vi "High Throughput Streaming (FPGA) PXIe-796xR.vi"() -> ()   [LabVIEW 2016]
doc: "Example Description:\nThis FPGA VI has two data streaming engines. One to stream data to disk from the FPGA and one to stream data from disk to the FPGA. The throughput of the streams is controled by accessing the DMA FIFOs on a subset of the cycles of the SCTLs.\n\nRunning the VI:\nThis VI m ust be run from one of the High Throughput Streaming - XXXXXXX (Host).vi files in the project. Refer to the host documentation for steps regarding running and configuring this FPGA VI.\n\nExecution Steps:\nRefer to teh block diagram of this VI for excution comments."
uses:
  <vilib>/Platform/TimedLoop/XDataNode/timing_clust.ctl
  <vilib>/Platform/TimedLoop/XDataNode/nitl_modes.ctl
  <vilib>/Platform/TimedLoop/XDataNode/wakeup.ctl
  <vilib>/rvi/Emulation/niFpgaGetClockAttributes.vi
  <vilib>/rvi/Emulation/niFpgaSctlEmulationGetInTimedLoop.vi
  <vilib>/rvi/Emulation/niFpgaEmulationReportErrorSimple.vi
  <vilib>/rvi/Emulation/niFpgaCriticalErrorInLSC.vi
  <vilib>/rvi/interface/RandomDataEmulation/nirviRandomDataMultiElementFPGAFIFO.vi
  <instcachedir>/0/nirviRandomDataMultiElementFPGAFIFO_6740B454F3C245F78F76ED91F73FD8DB.lvgen/nirviRandomDataMultiElementFPGAFIFO_6740B454F3C245F78F76ED91F73FD8DB_001.vi
  <vilib>/rvi/interface/RandomDataEmulation/niFpgaRandomDataHandleErrors.vi
  <vilib>/Platform/TimedLoop/XDataNode/XDataNode.xnode
  <vilib>/rvi/DataTransferAndStorage/Container/XNode/niFpgaContainer.xnode
  <vilib>/rvi/interface/RandomDataEmulation/nirviRandomDataFpgaMultiElementTemplate.vi
  <vilib>/Platform/TimedLoop/XDataNode/XDNodeRunTimeDep.lvlib
panel:
  in  "output.Requested Throughput Denominator":u16=200
  in  "input.Requested Throughput Denominator":u16=200
  out "input.Max Throughput":u16
  in  "input.Requested Throughput":u16
  out "input.FIFO Transfer Status":T1
  in  "output.Requested Throughput":u16
  out "output.Max Throughput":u16
  out "output.FIFO Transfer Status":T2
  in  "output.Start":bool
  out "output.Ever Timed Out?":bool
  in  "output.Reset":bool
  out "output.Number of Elements to Read":u32
  out "output.Minimum Number of Elements to Read":u32
  out "output.FIFO Size":u32
  in  "output.Stop":bool
  in  "input.Stop":bool
  in  "input.Start":bool
  out "input.FIFO Size":u32
  out "input.Minimum Number of Elements to Write":u32
  out "input.Number of Elements to Write":u32
  in  "input.Reset":bool
  out "input.Ever Timed Out?":bool
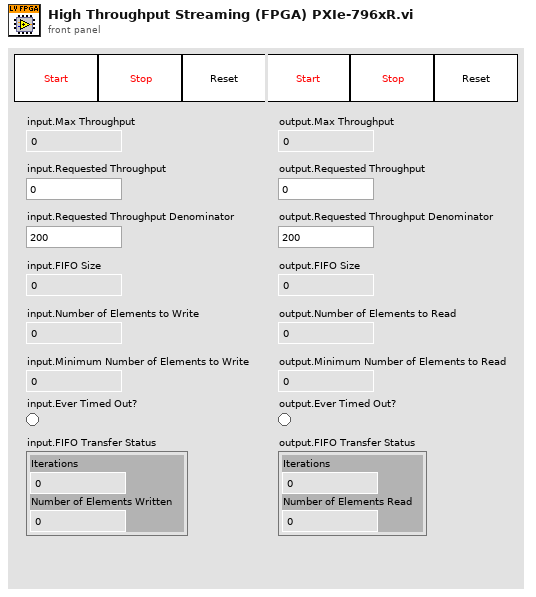
[diagram p1: front panel]
types:
  T1 = cluster{"Iterations":u64, "Number of Elements Written":u64}
  T2 = cluster{"Iterations":u64, "Number of Elements Read":u64}
  T3 = typedef "XDNodeRunTimeDep.lvlib/timing_clust.ctl" = cluster{"Expected End [f-1]":u64, "Actual End [f-1]":u64, "Finished Late? [f-1]":bool, "Expected End [i-1]":u64, "Actual End [i-1]":u64, "Finished Late? [i-1]":bool, "Expected Start [i]":u64, "Actual Start [i]":u64, "Expected Start [f]":u64, "Actual Start [f]":u64, "Source Name":string, "Structure Name":string, "Period":i64, "Deadline":i64, "Offset":i64, "Start":i64, "Priority":i32, "Timeout":i32, "Mode":T4, "Wakeup Reason":T5, "Error":errorcluster, "Source Type":string, "Secondary Source Type":string, "Global End Time":u64, "Global Start Time":u64, "Frame Duration":u64, "Iteration Duration":u64, "Assigned CPU":i32, "I/O Scan Engine Mode":u32}
  T4 = typedef "XDNodeRunTimeDep.lvlib/nitl_modes.ctl" = enum32{"No Change", "Process missed periods, maintain original phase", "Discard missed periods, maintain original phase", "Process missed periods, ignore original phase", "Discard missed periods, ignore original phase"}
  T5 = typedef "XDNodeRunTimeDep.lvlib/wakeup.ctl" = enum32{"Normal", "Aborted", "Asynchronous wakeup", "Timing source error", "Timed loop error", "Timeout"}
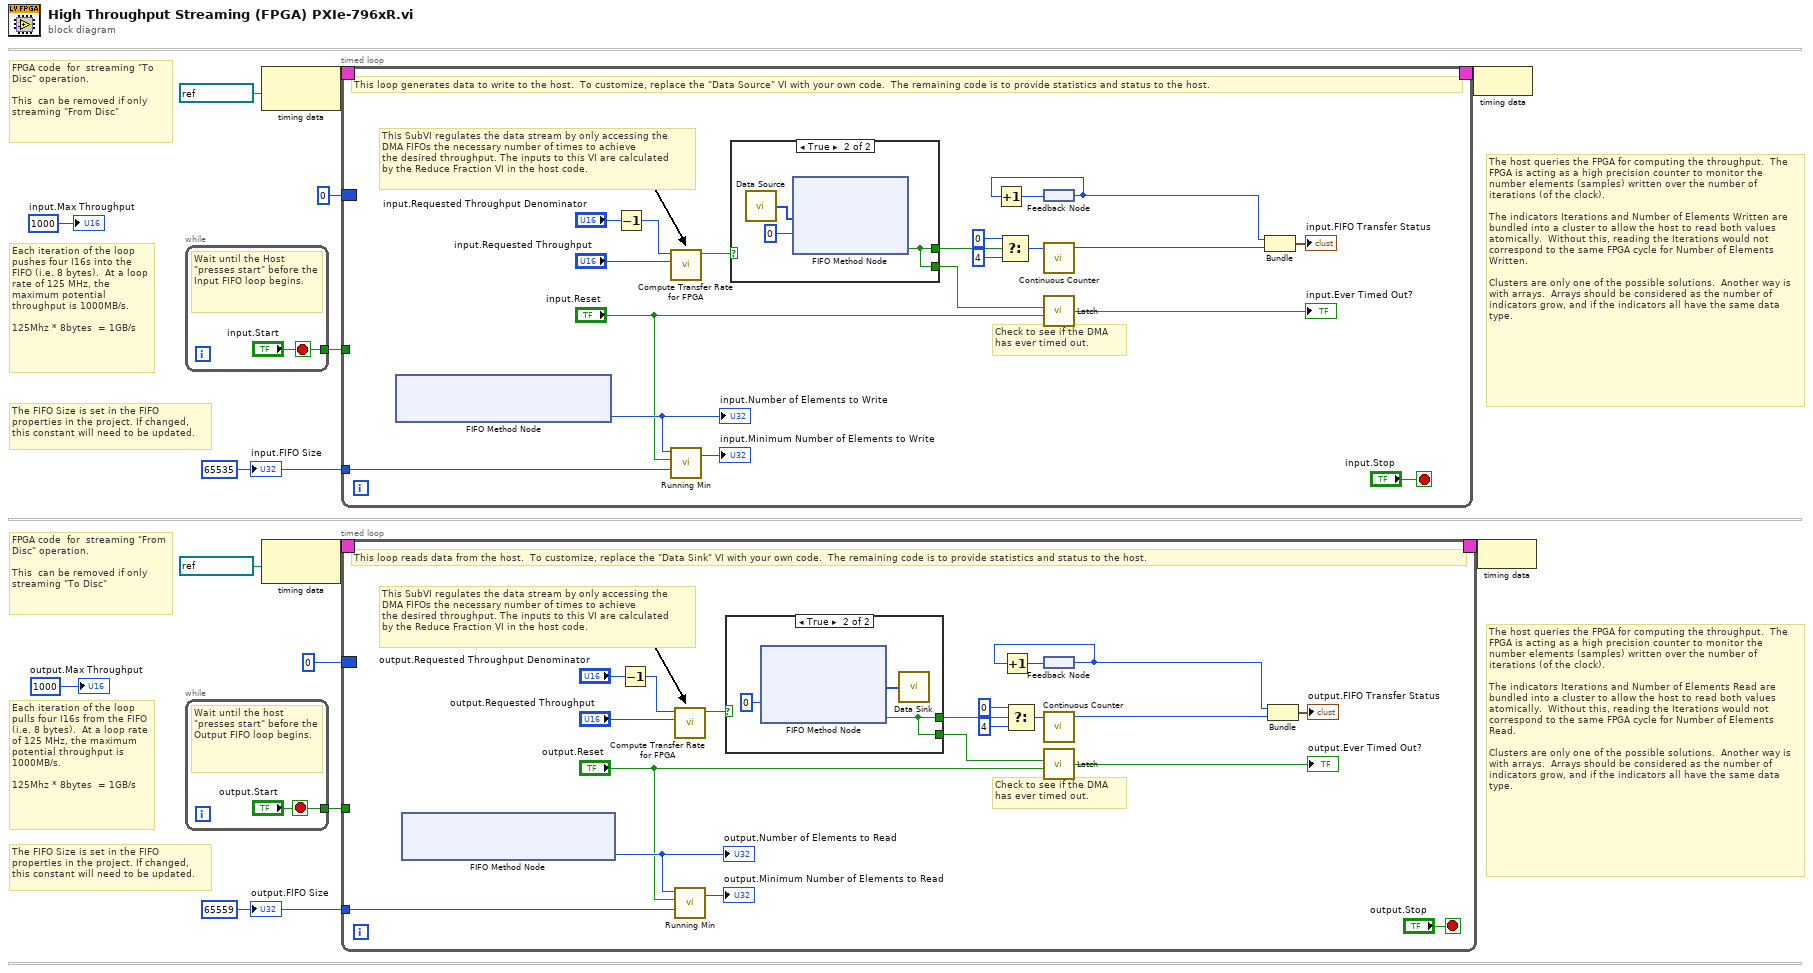
[diagram p0: block diagram]
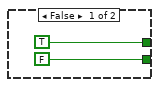
[diagram p2: hidden frame]
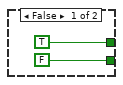
[diagram p3: hidden frame]
diagram:
  w5 = u32 65559 ("output.FIFO Size")
  w2 = u32 65535 ("input.FIFO Size")
  # "The FIFO Size is set in the FIFO\nproperties in the project. If changed, \nthis constant will need to be updated."
  # "The FIFO Size is set in the FIFO\nproperties in the project. If changed, \nthis constant will need to be updated."
  # "FPGA code  for  streaming \"To Disc\" operation. \n\nThis  can be removed if only streaming \"From Disc\""
  # "FPGA code  for  streaming \"From Disc\" operation. \n\nThis  can be removed if only streaming \"To Disc\""
  # "Each iteration of the loop pulls four I16s from the FIFO (i.e. 8 bytes).  At a loop rate of 125 MHz, the maximum potential throughput is 1000MB/s.\n\n125Mhz * 8bytes  = 1GB/s"
  # "The host queries the FPGA for computing the throughput.  The FPGA is acting as a high precision counter to monitor the number elements (samples) written over the number of iterations (of the clock).\n\nThe indicators Iterations and Number of Elements Read are bundled into a cluster to allow the host to read both values atomically.  Without this, reading the Iterations would not correspond to the same FPGA cycle for Number of Elements Read.\n\nClusters are only one of the possible solutions.  Another way is with arrays.  Arrays should be considered as the number of indicators grow, and if the indicators all have the same data type."
  # "Each iteration of the loop pushes four I16s into the FIFO (i.e. 8 bytes).  At a loop rate of 125 MHz, the maximum potential throughput is 1000MB/s.\n\n125Mhz * 8bytes  = 1GB/s"
  # "The host queries the FPGA for computing the throughput.  The FPGA is acting as a high precision counter to monitor the number elements (samples) written over the number of iterations (of the clock).\n\nThe indicators Iterations and Number of Elements Written are bundled into a cluster to allow the host to read both values atomically.  Without this, reading the Iterations would not correspond to the same FPGA cycle for Number of Elements Written.\n\nClusters are only one of the possible solutions.  Another way is with arrays.  Arrays should be considered as the number of indicators grow, and if the indicators all have the same data type."
  n1 = while {
    tunnel: ["input.Start"] -> w11
    stop <- "input.Start" stop-if-true
    # "Wait until the Host \"presses start\" before the Input FIFO loop begins."
  }
  n2 = while {
    tunnel: ["output.Start"] -> w8
    stop <- "output.Start" stop-if-true
    # "Wait until the host \"presses start\" before the Output FIFO loop begins."
  }
  n3 = node-c288(refnum<k21> "125 MHz" ("Source Name")) -> (w14:T3)
  n4 = node-c288(refnum<k21> "125 MHz" ("Source Name")) -> (w10:T3)
  n5 = timed-loop {
    timing: w14 -> [_]
    timing-out: [_] -> w13
    tunnel: w11 -> [_]
    tunnel: w2 -> [w35]
    border: u64 0 -> [_]
    stop <- "input.Stop" stop-if-true
    # "Check to see if the DMA \nhas ever timed out."
    # "This SubVI regulates the data stream by only accessing the \nDMA FIFOs the necessary number of times to achieve \nthe desired throughput. The inputs to this VI are calculated \nby the Reduce Fraction VI in the host code."
    # "This loop generates data to write to the host.  To customize, replace the \"Data Source\" VI with your own code.  The remaining code is to provide statistics and status to the host."
    n6 = xnode ("FIFO Method Node")() -> ("Number of Elements to Write"=w32:u32)  [unwired: 1 in, 1 out]
    "input.Number of Elements to Write" <- w32
    n7 = Decrement(x="input.Requested Throughput Denominator") -> (x-1=w18:u16)
    n8 = call "Compute Transfer Rate for FPGA.vi"("Duty Rate"="input.Requested Throughput", "Clock Rate (minus 1)"=w18) -> ("Output"=w21:bool)  [unwired: 4 in, 1 out]
    n9 = call "Running Min.vi"("Starting Min"=w35, "Reset"="input.Reset", "Next Value"=w32) -> ("Running Min"=→"input.Minimum Number of Elements to Write":u32)  [unwired: 4 in]
    n10 = case shown="True" w21 {
      tunnel: [TRUE ("Timed Out?") w38] -> w20
      tunnel: [FALSE ("Timed Out?") w38] -> w19
      frame False {
      }
      frame True {
        n11 = call "Data Source.vi"() -> ("Elements"=w39:i16[])
        n12 = xnode ("FIFO Method Node")("Element"=w39, "Timeout"=0) -> ("Timed Out?"=w38:bool)  [unwired: 1 in, 1 out]
      }
    }
    n13 = Select(t=u8 0, s=w20, f=u8 4) -> (s? t:f=w29:u8)
    n14 = feedback #1() -> (w26:u64)
    n15 = Increment(x=w26) -> (x+1=w27:u64)
    n16 = feedback-in #1(w27) -> ()
    n17 = call "Continuous Counter.vi"("value"=w29) -> ("count"=w25:u64)  [unwired: 6 in]
    n18 = call <vilib>:"Latch.vi"("Clear"="input.Reset", "Set"=w19) -> ("Output"=→"input.Ever Timed Out?":bool)  [unwired: 4 in]
    n19 = Bundle(w26, "count"=w25) -> (→"input.FIFO Transfer Status":cluster{u64, "count":u64})  [unwired: 1 in]
  }
  n20 = timed-loop {
    timing: w10 -> [_]
    timing-out: [_] -> w9
    tunnel: w8 -> [_]
    border: u64 0 -> [_]
    tunnel: w5 -> [w51]
    stop <- "output.Stop" stop-if-true
    # "Check to see if the DMA \nhas ever timed out."
    # "This SubVI regulates the data stream by only accessing the \nDMA FIFOs the necessary number of times to achieve \nthe desired throughput. The inputs to this VI are calculated \nby the Reduce Fraction VI in the host code."
    # "This loop reads data from the host.  To customize, replace the \"Data Sink\" VI with your own code.  The remaining code is to provide statistics and status to the host."
    n21 = xnode ("FIFO Method Node")() -> ("Number of Elements to Read"=w60:u32)  [unwired: 1 in, 1 out]
    "output.Number of Elements to Read" <- w60
    n22 = Decrement(x="output.Requested Throughput Denominator") -> (x-1=w44:u16)
    n23 = call "Compute Transfer Rate for FPGA.vi"("Duty Rate"="output.Requested Throughput", "Clock Rate (minus 1)"=w44) -> ("Output"=w47:bool)  [unwired: 4 in, 1 out]
    n24 = call "Running Min.vi"("Starting Min"=w51, "Reset"="output.Reset", "Next Value"=w60) -> ("Running Min"=→"output.Minimum Number of Elements to Read":u32)  [unwired: 4 in]
    n25 = case shown="True" w47 {
      tunnel: [TRUE ("Timed Out?") w64] -> w53
      tunnel: [FALSE ("Timed Out?") w64] -> w45
      frame False {
      }
      frame True {
        n26 = xnode ("FIFO Method Node")("Timeout"=0) -> ("Element"=w65:i16[], "Timed Out?"=w64:bool)  [unwired: 1 in, 1 out]
        n27 = call "Data Sink.vi"("Elements"=w65) -> ()
      }
    }
    n28 = Select(t=u8 0, s=w53, f=u8 4) -> (s? t:f=w56:u8)
    n29 = feedback #2() -> (w50:u64)
    n30 = Increment(x=w50) -> (x+1=w58:u64)
    n31 = feedback-in #2(w58) -> ()
    n32 = call "Continuous Counter.vi"("value"=w56) -> ("count"=w49:u64)  [unwired: 6 in]
    n33 = call <vilib>:"Latch.vi"("Clear"="output.Reset", "Set"=w45) -> ("Output"=→"output.Ever Timed Out?":bool)  [unwired: 4 in]
    n34 = Bundle(w50, "count"=w49) -> (→"output.FIFO Transfer Status":cluster{u64, "count":u64})  [unwired: 1 in]
  }
  n35 = node-c288(w13) -> ()
  n36 = node-c288(w9) -> ()
  "input.FIFO Size" <- w2
  "output.FIFO Size" <- w5
  "output.Max Throughput" <- u16 1000 ("output.Max Throughput")
  "input.Max Throughput" <- u16 1000 ("input.Max Throughput")
